vi "array for loop.vi"() -> ()   [LabVIEW 2017]
panel:
  out "Numeric":i32
  out "Array 2":string[](array[string])
  out "Array 4":bool[](array[boolean])
  out "Array":dbl[](array[numeric])
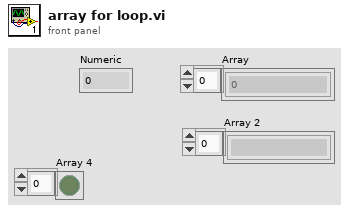
[diagram p1: front panel]
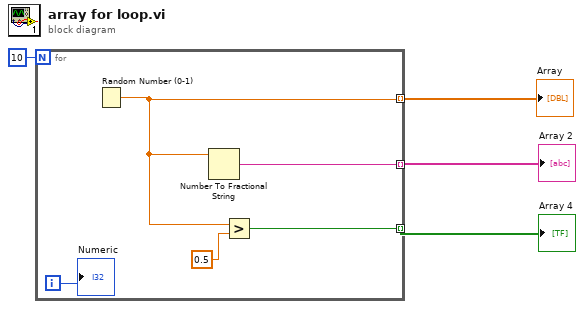
[diagram p0: block diagram]
diagram:
  n1 = for {
    N: 10 -> [_]
    tunnel: [w8] -> w3 mode=indexing
    tunnel: [w7] -> w2 mode=indexing
    tunnel: [w6] -> w1 mode=indexing
    i -> [w5]
    n2 = Random Number (0-1)() -> (number: 0 to 1=w8:dbl)
    n3 = Number To Fractional String(number=w8) -> (F-format string=w6:string)  [unwired: 3 in]
    n4 = Greater?(x=w8, y=0.5) -> (0:w7:bool)
    "Numeric" <- w5
  }
  "Array" <- w3
  "Array 4" <- w2
  "Array 2" <- w1
